vi "setSquareParameters.vi"(11 "square in":T1) -> (2 "Match":bool, 3 "square out":T1)   [LabVIEW 2020]
uses:
  Global Variables/Global Number of Indices.vi
  Global Variables/Global Difficulty Level.vi
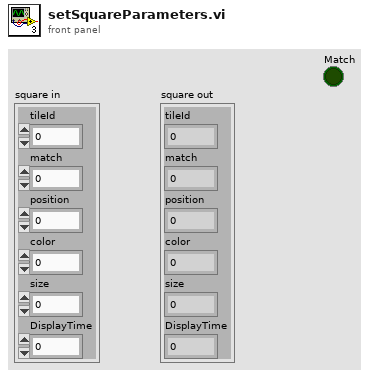
[diagram p1: front panel]
types:
  T1 = cluster{"tileId":i32, "match":i32, "position":i32, "color":u32, "size":i32, "DisplayTime":i32}
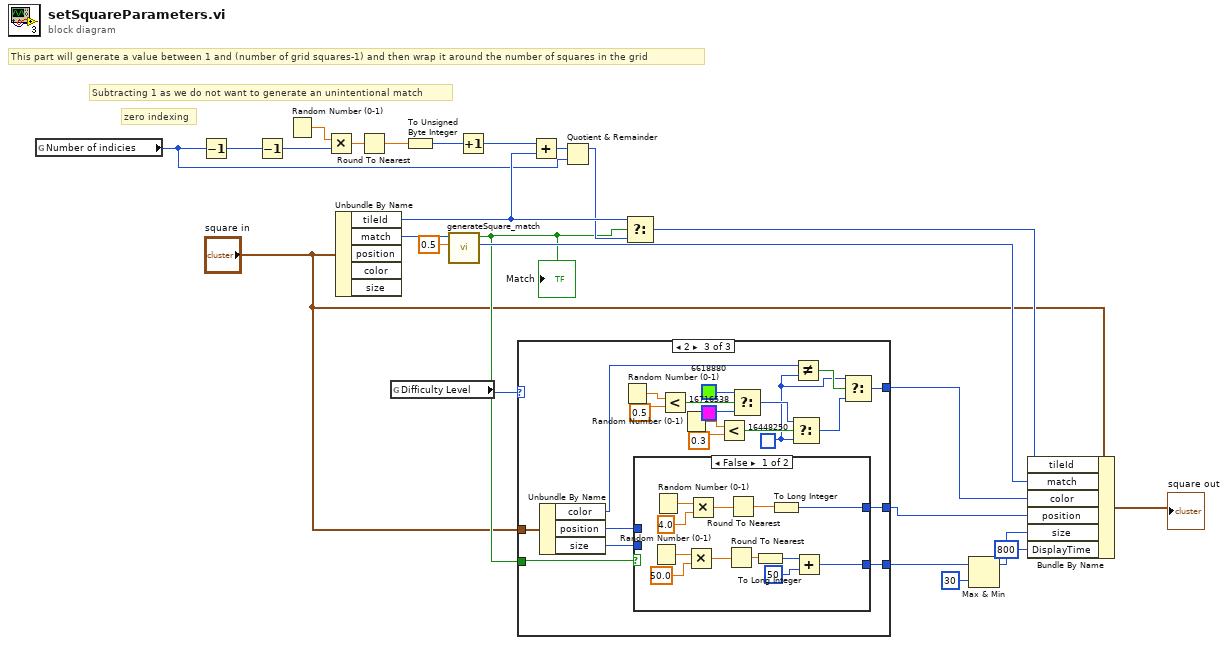
[diagram p0: block diagram]
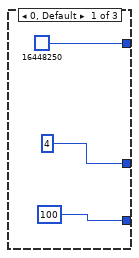
[diagram p2: hidden frame]
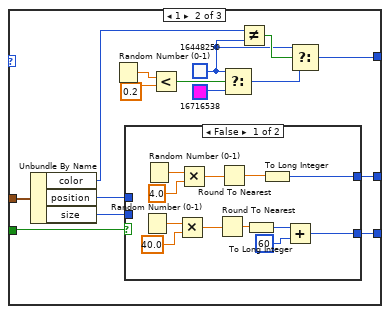
[diagram p3: hidden frame]
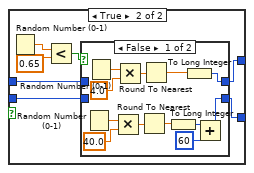
[diagram p4: hidden frame]
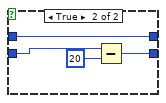
[diagram p5: hidden frame]
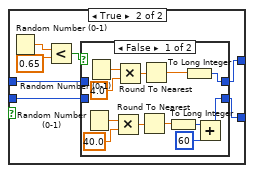
[diagram p6: hidden frame]
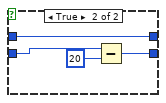
[diagram p7: hidden frame]
diagram:
  # "zero indexing"
  # "This part will generate a value between 1 and (number of grid squares-1) and then wrap it around the number of squares in the grid"
  # "Subtracting 1 as we do not want to generate an unintentional match"
  n1 = global read "Global Number of Indices.vi" "Number of indicies"() -> (w17:u8)
  n2 = Decrement(x=w17) -> (x-1=w16:u8)
  n3 = Decrement(x=w16) -> (x-1=w13:u8)
  n4 = Random Number (0-1)() -> (number: 0 to 1=w10:dbl)
  n5 = Multiply(x=w10, y=w13) -> (x*y=w11:dbl)
  n6 = Unbundle By Name("square in") -> ("tileId"=w25:i32, "match"=w19:i32)  [unwired: 3 out]
  n7 = Round To Nearest(number=w11) -> (nearest integer value=w12:dbl)
  n8 = global read "Global Difficulty Level.vi" "Difficulty Level"() -> (w9:u8)
  n9 = To Unsigned Byte Integer(number=w12) -> (unsigned 8bit integer=w15:u8)
  n10 = call "generateSquare_match.vi"("Match rate (0-1)"=sgl 0.5, "match"=w19) -> ("new match"=w21:i32, "Match"=w8:bool)  [unwired: 6 in]
  "Match" <- w8
  n11 = Increment(x=w15) -> (x+1=w24:u8)
  n12 = case shown="2" w9 {
    tunnel: [4 w32 w88] -> w6
    tunnel: [u32 16448250 w34 w90] -> w7
    tunnel: [100 w31 w87] -> w5
    tunnel: w8 -> [_ w33 w89]
    tunnel: "square in" -> [_ w39 w94]
    frame 0, Default {
    }
    frame 1 {
      w36 = u32 16448250
      n13 = Unbundle By Name(w39) -> ("color"=w37:u32, "position"=w30:i32, "size"=w29:i32)
      n14 = Random Number (0-1)() -> (number: 0 to 1=w43:dbl)
      n15 = case shown="False" w33 {
        tunnel: [w51 w58] -> w32
        tunnel: [w44 w56] -> w31
        tunnel: w30 -> [_ w59]
        tunnel: w29 -> [_ w57]
        frame False {
          n16 = Random Number (0-1)() -> (number: 0 to 1=w50:dbl)
          n17 = Random Number (0-1)() -> (number: 0 to 1=w55:dbl)
          n18 = Multiply(x=w50, y=40.0) -> (x*y=w48:dbl)
          n19 = Multiply(x=w55, y=4.0) -> (x*y=w53:dbl)
          n20 = Round To Nearest(number=w48) -> (nearest integer value=w47:dbl)
          n21 = Round To Nearest(number=w53) -> (nearest integer value=w52:dbl)
          n22 = To Long Integer(number=w47) -> (32bit integer=w46:i32)
          n23 = To Long Integer(number=w52) -> (32bit integer=w51:i32)
          n24 = Add(x=w46, y=60) -> (x+y=w44:i32)
        }
        frame True {
          n25 = Random Number (0-1)() -> (number: 0 to 1=w62:dbl)
          n26 = Less?(x=w62, y=0.65) -> (x < y?=w60:bool)
          n27 = case shown="False" w60 {
            tunnel: w59 -> [_ w78]
            tunnel: [w64 w78] -> w58
            tunnel: w57 -> [_ w76]
            tunnel: [w63 w77] -> w56
            frame False {
              n28 = Random Number (0-1)() -> (number: 0 to 1=w70:dbl)
              n29 = Random Number (0-1)() -> (number: 0 to 1=w74:dbl)
              n30 = Multiply(x=w70, y=40.0) -> (x*y=w68:dbl)
              n31 = Multiply(x=w74, y=4.0) -> (x*y=w72:dbl)
              n32 = Round To Nearest(number=w68) -> (nearest integer value=w67:dbl)
              n33 = Round To Nearest(number=w72) -> (nearest integer value=w71:dbl)
              n34 = To Long Integer(number=w67) -> (32bit integer=w66:i32)
              n35 = To Long Integer(number=w71) -> (32bit integer=w64:i32)
              n36 = Add(x=w66, y=60) -> (x+y=w63:i32)
            }
            frame True {
              n37 = Subtract(x=w76, y=20) -> (x-y=w77:i32)
            }
          }
        }
      }
      n38 = Less?(x=w43, y=0.2) -> (x < y?=w41:bool)
      n39 = Select(t=w36, s=w41, f=u32 16716538) -> (s? t:f=w35:u32)
      n40 = Not Equal?(x=w37, y=w36) -> (x != y?=w38:bool)
      n41 = Select(t=w36, s=w38, f=w35) -> (s? t:f=w34:u32)
    }
    frame 2 {
      w79 = u32 16448250
      n42 = Unbundle By Name(w94) -> ("color"=w92:u32, "position"=w86:i32, "size"=w85:i32)
      n43 = Random Number (0-1)() -> (number: 0 to 1=w98:dbl)
      n44 = case shown="False" w89 {
        tunnel: [w106 w113] -> w88
        tunnel: [w99 w111] -> w87
        tunnel: w86 -> [_ w114]
        tunnel: w85 -> [_ w112]
        frame False {
          n45 = Random Number (0-1)() -> (number: 0 to 1=w105:dbl)
          n46 = Random Number (0-1)() -> (number: 0 to 1=w110:dbl)
          n47 = Multiply(x=w105, y=50.0) -> (x*y=w103:dbl)
          n48 = Multiply(x=w110, y=4.0) -> (x*y=w108:dbl)
          n49 = Round To Nearest(number=w103) -> (nearest integer value=w102:dbl)
          n50 = Round To Nearest(number=w108) -> (nearest integer value=w107:dbl)
          n51 = To Long Integer(number=w102) -> (32bit integer=w101:i32)
          n52 = To Long Integer(number=w107) -> (32bit integer=w106:i32)
          n53 = Add(x=w101, y=50) -> (x+y=w99:i32)
        }
        frame True {
          n54 = Random Number (0-1)() -> (number: 0 to 1=w117:dbl)
          n55 = Less?(x=w117, y=0.65) -> (x < y?=w115:bool)
          n56 = case shown="False" w115 {
            tunnel: w114 -> [_ w133]
            tunnel: [w119 w133] -> w113
            tunnel: w112 -> [_ w131]
            tunnel: [w118 w132] -> w111
            frame False {
              n57 = Random Number (0-1)() -> (number: 0 to 1=w125:dbl)
              n58 = Random Number (0-1)() -> (number: 0 to 1=w129:dbl)
              n59 = Multiply(x=w125, y=40.0) -> (x*y=w123:dbl)
              n60 = Multiply(x=w129, y=4.0) -> (x*y=w127:dbl)
              n61 = Round To Nearest(number=w123) -> (nearest integer value=w122:dbl)
              n62 = Round To Nearest(number=w127) -> (nearest integer value=w126:dbl)
              n63 = To Long Integer(number=w122) -> (32bit integer=w121:i32)
              n64 = To Long Integer(number=w126) -> (32bit integer=w119:i32)
              n65 = Add(x=w121, y=60) -> (x+y=w118:i32)
            }
            frame True {
              n66 = Subtract(x=w131, y=20) -> (x-y=w132:i32)
            }
          }
        }
      }
      n67 = Less?(x=w98, y=0.5) -> (x < y?=w96:bool)
      n68 = Random Number (0-1)() -> (number: 0 to 1=w84:dbl)
      n69 = Less?(x=w84, y=0.3) -> (x < y?=w82:bool)
      n70 = Select(t=u32 6618880, s=w96, f=u32 16716538) -> (s? t:f=w81:u32)
      n71 = Select(t=w81, s=w82, f=w79) -> (s? t:f=w80:u32)
      n72 = Not Equal?(x=w92, y=w79) -> (x != y?=w93:bool)
      n73 = Select(t=w79, s=w93, f=w80) -> (s? t:f=w90:u32)
    }
  }
  n74 = Add(x=w24, y=w25) -> (x+y=w14:i32)
  n75 = Quotient & Remainder(x=w14, y=w17) -> (x-y*floor(x/y)=w18:i32)  [unwired: 1 out]
  n76 = Select(t=w25, s=w8, f=w18) -> (s? t:f=w22:i32)
  n77 = Max & Min(x=w5, y=30) -> (max(x,y)=w3:i32)  [unwired: 1 out]
  n78 = Bundle By Name(cluster="square in", "tileId"=w22, "match"=w21, "color"=w7, "position"=w6, "size"=w3, "DisplayTime"=800) -> (→"square out":T1)
